vi "FilterStringProperties.vi"(11 "properties":T1[](array[typedef]) {"data type" items=["Unknown"=0, "String"=23, "I32"=3, "I64"=4, "DBL"=10, "Time stamp"=30]; "object type" items=["File", "Channel Group", "Channel"]}) -> (3 "string properties":string[](array[string]))   [LabVIEW 2023]
doc: "Filters the given list of properties for all properties of data type string."
uses:
  <vilib>/DataFinder/DataTypes/property.ctl
  <vilib>/DataFinder/DataTypes/object type.ctl
  <vilib>/DataFinder/DataTypes/data type.ctl
  <vilib>/DataFinder/NI_DataFinder.lvlib
panel:
  # "From the list of indexed properties, filter only those with a data type string."
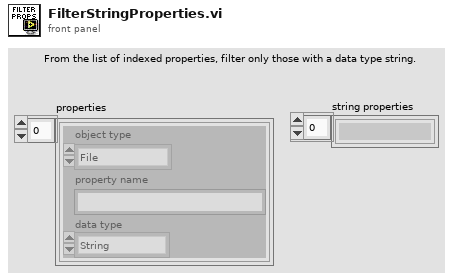
[diagram p1: front panel]
types:
  T1 = typedef "NI_DataFinder.lvlib/property.ctl" = cluster{"object type":T2, "property name":string, "data type":T3}
  T2 = typedef "NI_DataFinder.lvlib/object type.ctl" = u16
  T3 = typedef "NI_DataFinder.lvlib/data type.ctl" = u16
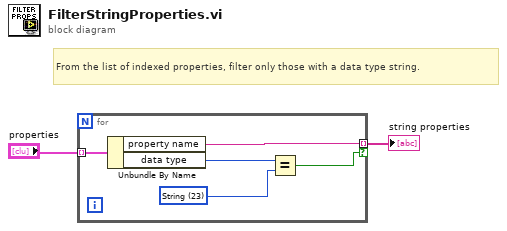
[diagram p0: block diagram]
diagram:
  # "From the list of indexed properties, filter only those with a data type string."
  n1 = for {
    tunnel: "properties" -> [w7] mode=indexing
    tunnel: [w5] -> w2 mode=indexing if=w4
    w3 = T3 23 items=["Unknown"=0, "String"=23, "I32"=3, "I64"=4, "DBL"=10, "Time stamp"=30] ("data type")
    n2 = Unbundle By Name(w7) -> ("property name"=w5:string, "data type"=w6:T3)
    n3 = Equal?(x=w6, y=w3) -> (x = y?=w4:bool)
  }
  "string properties" <- w2
